vi "Handle Incoming Packets.vi"(8 "error in (no error)":errorcluster, 9 "SessionMailbox":refnum<queue>, 10 "Incoming Packet":refnum<class "ControlPacket.lvclass">, 11 "Client in":refnum<class "Client.lvclass">) -> (0 "error out":errorcluster, 1 "SessionMailbox out":refnum<queue>, 2 "Outgoing":T1, 3 "Client out":refnum<class "Client.lvclass">)   [LabVIEW 2013, in "MQTT Server.lvlib" / "Client.lvclass"]
uses:
  Client.lvclass
  Control Packets/ControlPacket/ControlPacket.lvclass
  MQTT_Base/Response -- cluster.ctl
  Client.lvclass/Client.ctl
  Control Packets/CONNACK/CONNACK.lvclass
  Control Packets/CONNACK/Connect Return Code -- enum.ctl
  MQTT_Base/MQTT_Base.lvclass
  Control Packets/PUBREC/PUBREC.lvclass
  Control Packets/ControlPacket/ControlPacket.lvclass/ControlPacket.ctl
  Control Packets/PUBLISH/PUBLISH.lvclass
  Control Packets/PUBCOMP/PUBCOMP.lvclass
  Control Packets/SUBACK/SUBACK.lvclass
  Control Packets/UNSUBACK/UNSUBACK.lvclass
  Control Packets/PINGRESP/PINGRESP.lvclass
  Control Packets/PUBREL/PUBREL.lvclass
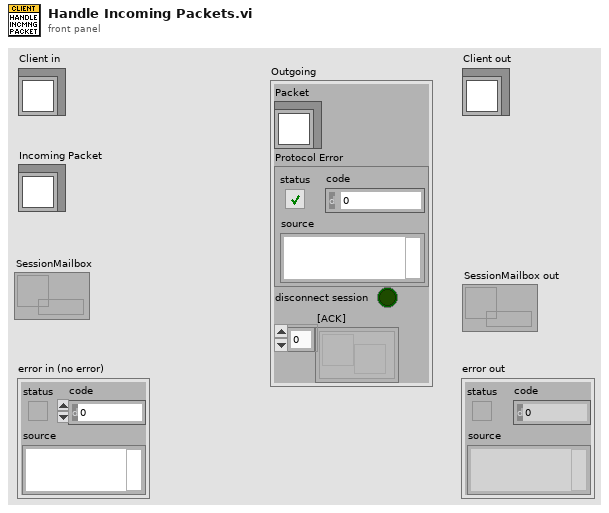
[diagram p1: front panel]
types:
  T1 = typedef "MQTT Server.lvlib/MQTT_Base.lvclass/Response -- cluster.ctl" = cluster{"Packet":refnum<class "ControlPacket.lvclass">, "Protocol Error":errorcluster, "disconnect session":bool, "[ACK]":refnum<notifier>[]}
  T2 = typedef "CONNACK.lvclass/Connect Return Code -- enum.ctl" = enum16{"Connection accepted", "Unacceptable protocol version", "Identifier Rejected", "Server Unavailable", "Bad Username or Password", "Not Authorized"}
  T3 = typedef "ControlPacket.lvclass/Control Packet Type -- enum.ctl" = enum16{"Reserved", "CONNECT", "CONNACK", "PUBLISH", "PUBACK", "PUBREC", "PUBREL", "PUBCOMP", "SUBSCRIBE", "SUBACK", "UNSUBSCRIBE", "UNSUBACK", "PINGREQ", "PINGRESP", "DISCONNECT", "Reserved(15)"}
  T4 = typedef "MQTT Server.lvlib/Client.lvclass/Public Events -- cluster.ctl" = cluster{"Connection Status":refnum<user-event>, "Connected":refnum<user-event>, "Application Message":refnum<user-event>}
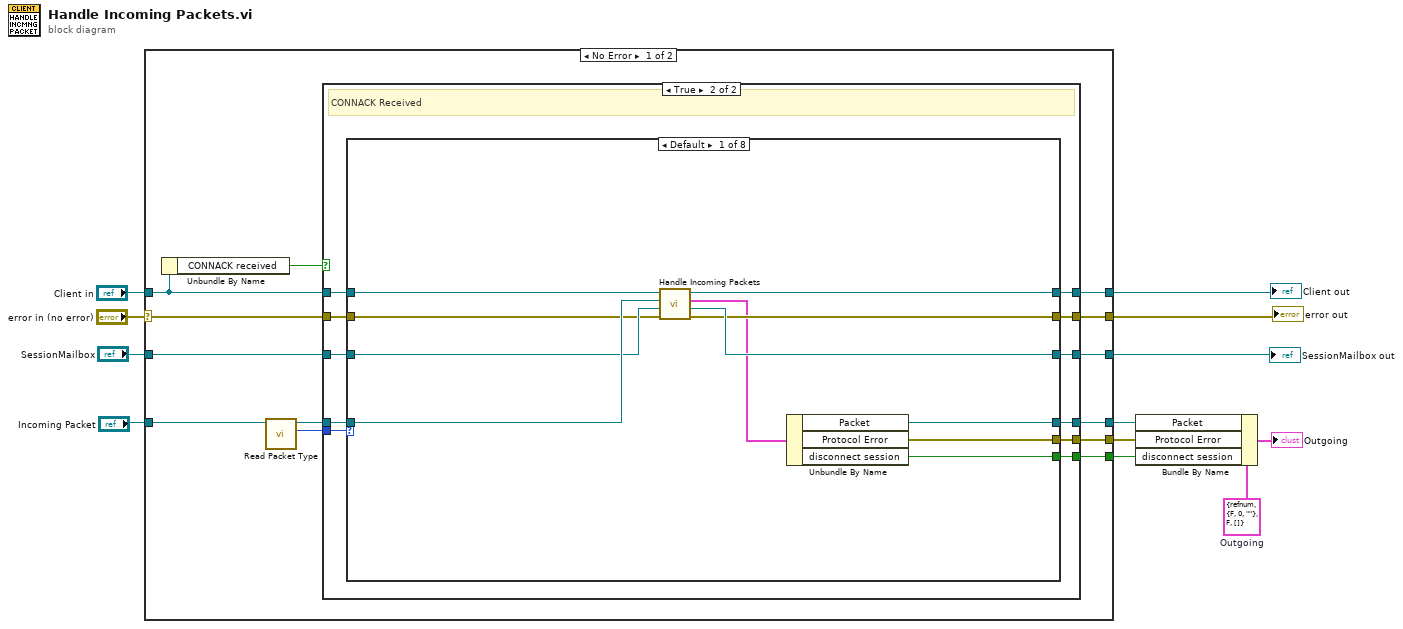
[diagram p0: block diagram]
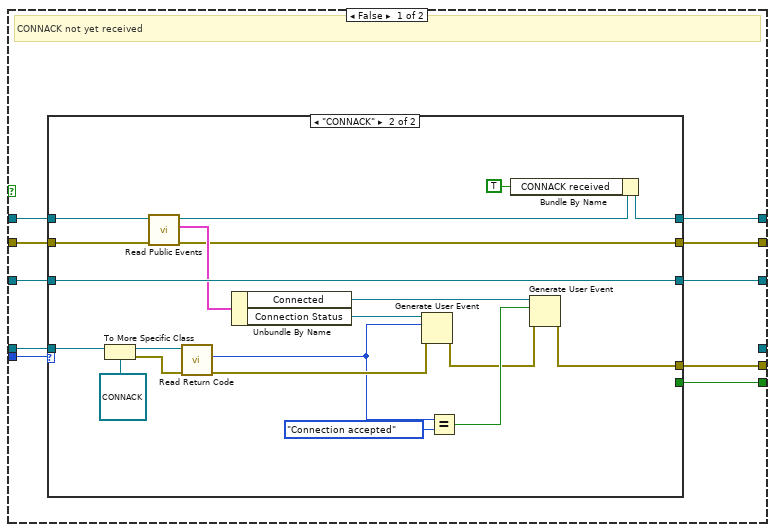
[diagram p2: hidden frame]
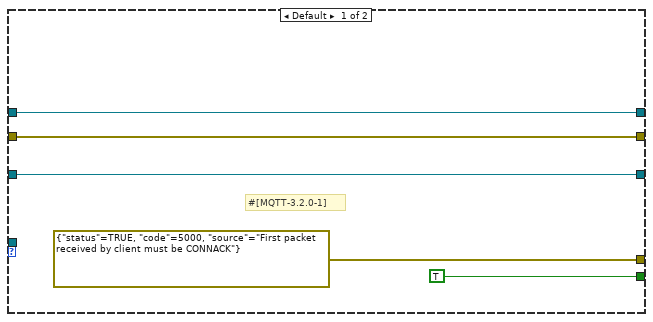
[diagram p3: hidden frame]
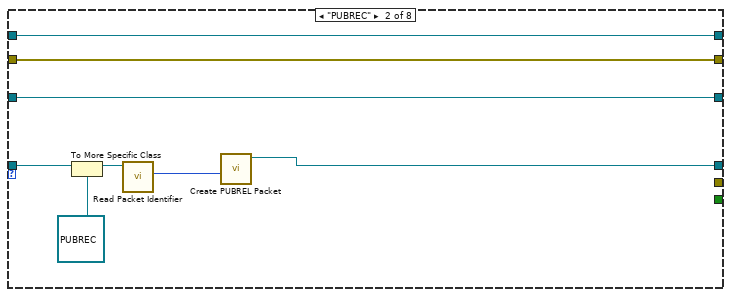
[diagram p4: hidden frame]
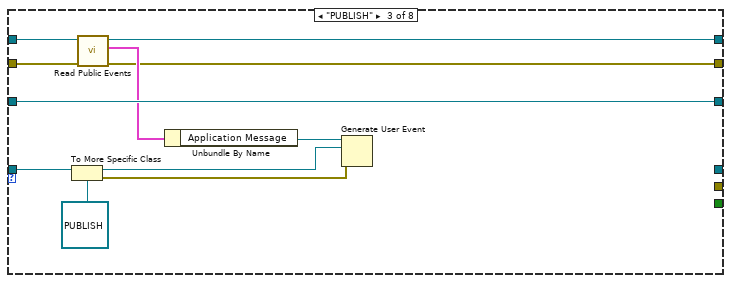
[diagram p5: hidden frame]
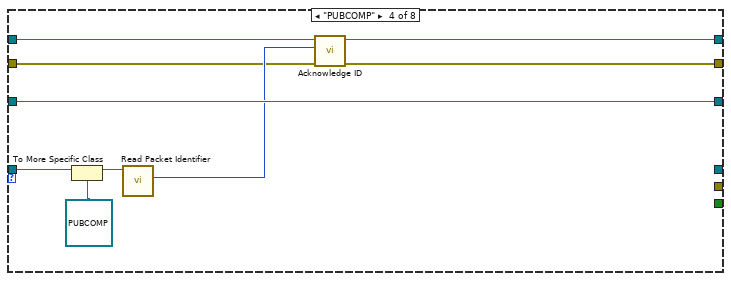
[diagram p6: hidden frame]
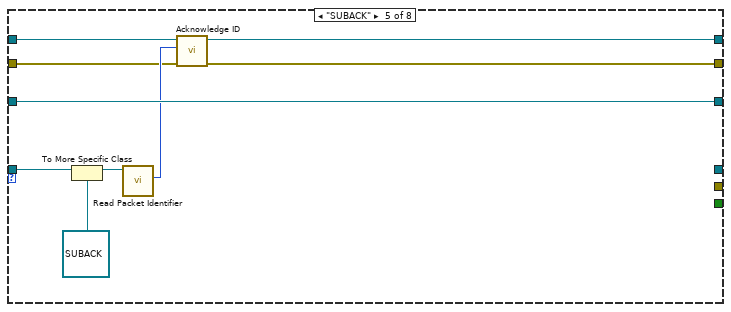
[diagram p7: hidden frame]
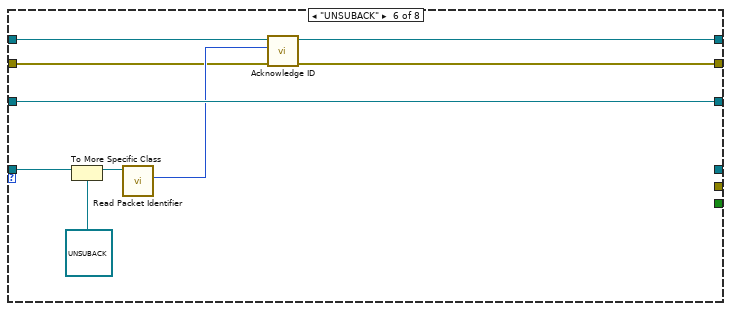
[diagram p8: hidden frame]
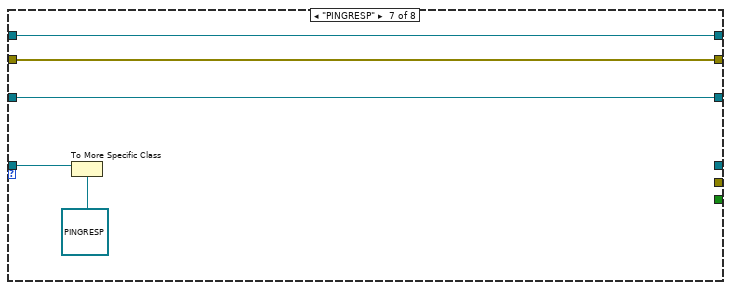
[diagram p9: hidden frame]
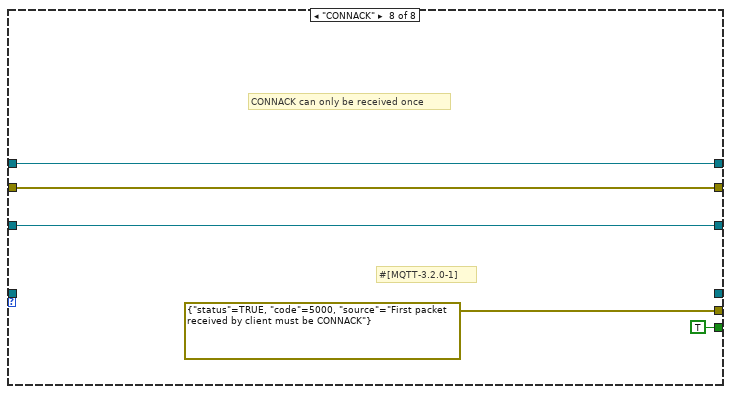
[diagram p10: hidden frame]
diagram:
  w12 = T1 {"Packet"=refnum, "Protocol Error"={"status"=FALSE, "code"=0, "source"=""}, "disconnect session"=FALSE, "[ACK]"=[]}  # Outgoing
  n1 = case shown="No Error" "error in (no error)" {
    selector: "error in (no error)" -> [w23 w141]
    tunnel: [w21 w141] -> w4
    tunnel: [w22 w140] -> w8
    tunnel: "Client in" -> [w14 w140]
    tunnel: "Incoming Packet" -> [w17 _]
    tunnel: [w20 _] -> w1
    tunnel: [w19 _] -> w10
    tunnel: "SessionMailbox" -> [w18 w139]
    tunnel: [w16 w139] -> w3
    tunnel: [w15 _] -> w11
    frame No Error {
      n2 = Unbundle By Name(w14) -> ("CONNACK received"=w13:bool)
      n3 = call "Read Packet Type.vi"("ControlPacket in"=w17) -> ("Control Packet Type"=w25:T3, "ControlPacket out"=w24:refnum<class "ControlPacket.lvclass">)  [unwired: 9 in]
      n4 = case shown="True" w13 {
        tunnel: w25 -> [w32 w71]
        tunnel: w24 -> [w35 w70]
        tunnel: w23 -> [w29 w69]
        tunnel: [w31 w68] -> w22
        tunnel: [w30 w67] -> w21
        tunnel: [_ w66] -> w20
        tunnel: [w34 w65] -> w19
        tunnel: w18 -> [w27 w64]
        tunnel: [w28 w63] -> w16
        tunnel: [w26 w62] -> w15
        tunnel: w14 -> [w33 w61]
        frame False {
          # "CONNACK not yet received"
          n5 = case shown="\"CONNACK\"" w32 {
            tunnel: w35 -> [_ w52]
            tunnel: [errorcluster {"status"=TRUE, "code"=5000, "source"="First packet received by client must be CONNACK"} ("error out 2") w51] -> w34
            tunnel: w33 -> [w40 w44]
            tunnel: [w40 w50] -> w31
            tunnel: [w39 w41] -> w30
            tunnel: w29 -> [w39 w42]
            tunnel: w27 -> [w38 w48]
            tunnel: [w38 w48] -> w28
            tunnel: [TRUE ("status") _] -> w26
            frame Default {
              # "#[MQTT-3.2.0-1]"
            }
            frame "CONNACK" {
              n6 = To More Specific Class(target class=refnum<class "CONNACK.lvclass"> refnum ("CONNACK in"), reference=w52) -> (specific class reference=w59:refnum<class "CONNACK.lvclass">, error out=w58:errorcluster)  [unwired: 1 in]
              n7 = call "Read Public Events.vi"("error in (no error)"=w42, "Client in"=w44) -> ("error out"=w41:errorcluster, "Client Public Events"=w47:T4, "Client out"=w43:refnum<class "Client.lvclass">)  [unwired: 7 in]
              n8 = call "Read Return Code.vi"("error in (no error)"=w58, "CONNACK in"=w59) -> ("error out"=w57:errorcluster, "Return Code"=w56:T2)  [unwired: 7 in, 1 out]
              n9 = Unbundle By Name(w47) -> ("Connected"=w46:refnum<user-event>, "Connection Status"=w45:refnum<user-event>)
              n10 = Generate User Event(user event=w45, event data cluster=w56, error in=w57) -> (error out=w53:errorcluster)  [unwired: 1 in, 1 out]
              n11 = Equal?(x=w56, y=Connect_Return_Code_--_enum."Connection accepted") -> (x = y?=w54:bool)
              n12 = Bundle By Name(cluster=w43, "CONNACK received"=TRUE) -> (w50:refnum<class "Client.lvclass">)
              n13 = Generate User Event(user event=w46, event data cluster=w54, error in=w53) -> (error out=w51:errorcluster)  [unwired: 1 in, 1 out]
            }
          }
        }
        frame True {
          # "CONNACK Received"
          n14 = case shown="Default" w71 {
            tunnel: w70 -> [w82 w87 w100 w109 w118 w127 w130 _]
            tunnel: w69 -> [w77 w89 w94 w103 w114 w121 w132 w138]
            tunnel: w61 -> [w79 w90 w92 w106 w112 w123 w133 w136]
            tunnel: [w78 w90 w91 w105 w111 w122 w133 w136] -> w68
            tunnel: [w76 w89 w93 w102 w113 w120 w132 w138] -> w67
            tunnel: w64 -> [w81 w88 w101 w110 w119 w128 w131 w137]
            tunnel: [w74 w83 _ _ _ _ _ _] -> w66
            tunnel: [w73 _ _ _ _ _ _ errorcluster {"status"=TRUE, "code"=5000, "source"="First packet received by client must be CONNACK"} ("error out 2")] -> w65
            tunnel: [w80 w88 w101 w110 w119 w128 w131 w137] -> w63
            tunnel: [w72 _ _ _ _ _ _ TRUE ("disconnect")] -> w62
            frame Default {
              n15 = call-parent "Handle Incoming Packets.vi"("error in (no error)"=w77, "SessionMailbox"=w81, "Incoming Packet"=w82, "MQTT_Base in"=w79) -> ("error out"=w76:errorcluster, "SessionMailbox out"=w80:refnum<queue>, "Outgoing"=w75:T1, "MQTT_Base out"=w78:refnum<class "Client.lvclass">)  [unwired: 4 in]
              n16 = Unbundle By Name(w75) -> ("Packet"=w74:refnum<class "ControlPacket.lvclass">, "Protocol Error"=w73:errorcluster, "disconnect session"=w72:bool)
            }
            frame "PUBREC" {
              n17 = To More Specific Class(target class=refnum<class "PUBREC.lvclass"> refnum ("PUBREC.lvclass"), reference=w87) -> (specific class reference=w85:refnum<class "PUBREC.lvclass">)  [unwired: 1 in, 1 out]
              n18 = call "Read Packet Identifier.vi"("ControlPacket in"=w85) -> ("Packet Identifier"=w84:u16)  [unwired: 9 in, 1 out]
              n19 = call "Create PUBREL Packet.vi"("Packet ID"=w84) -> ("PUBREL out"=w83:refnum<class "PUBREL.lvclass">)  [unwired: 9 in, 1 out]
            }
            frame "PUBLISH" {
              n20 = To More Specific Class(target class=refnum<class "PUBLISH.lvclass"> refnum ("PUBLISH.lvclass"), reference=w100) -> (specific class reference=w96:refnum<class "PUBLISH.lvclass">, error out=w95:errorcluster)  [unwired: 1 in]
              n21 = call "Read Public Events.vi"("error in (no error)"=w94, "Client in"=w92) -> ("error out"=w93:errorcluster, "Client Public Events"=w98:T4, "Client out"=w91:refnum<class "Client.lvclass">)  [unwired: 7 in]
              n22 = Unbundle By Name(w98) -> ("Application Message"=w97:refnum<user-event>)
              n23 = Generate User Event(user event=w97, event data cluster=w96, error in=w95) -> ()  [unwired: 1 in, 2 out]
            }
            frame "PUBCOMP" {
              n24 = To More Specific Class(target class=refnum<class "PUBCOMP.lvclass"> refnum ("PUBCOMP.lvclass"), reference=w109) -> (specific class reference=w108:refnum<class "PUBCOMP.lvclass">)  [unwired: 1 in, 1 out]
              n25 = call "Read Packet Identifier.vi"("ControlPacket in"=w108) -> ("Packet Identifier"=w104:u16)  [unwired: 9 in, 1 out]
              n26 = call "Acknowledge ID.vi"("error in (no error)"=w103, "Packet Identifier"=w104, "Client in"=w106) -> ("error out"=w102:errorcluster, "Client out"=w105:refnum<class "Client.lvclass">)  [unwired: 7 in]
            }
            frame "SUBACK" {
              n27 = To More Specific Class(target class=refnum<class "SUBACK.lvclass"> refnum ("SUBACK.lvclass"), reference=w118) -> (specific class reference=w117:refnum<class "SUBACK.lvclass">)  [unwired: 1 in, 1 out]
              n28 = call "Read Packet Identifier.vi"("ControlPacket in"=w117) -> ("Packet Identifier"=w115:u16)  [unwired: 9 in, 1 out]
              n29 = call "Acknowledge ID.vi"("error in (no error)"=w114, "Packet Identifier"=w115, "Client in"=w112) -> ("error out"=w113:errorcluster, "Client out"=w111:refnum<class "Client.lvclass">)  [unwired: 7 in]
            }
            frame "UNSUBACK" {
              n30 = To More Specific Class(target class=refnum<class "UNSUBACK.lvclass"> refnum ("UNSUBACK.lvclass"), reference=w127) -> (specific class reference=w126:refnum<class "UNSUBACK.lvclass">)  [unwired: 1 in, 1 out]
              n31 = call "Read Packet Identifier.vi"("ControlPacket in"=w126) -> ("Packet Identifier"=w124:u16)  [unwired: 9 in, 1 out]
              n32 = call "Acknowledge ID.vi"("error in (no error)"=w121, "Packet Identifier"=w124, "Client in"=w123) -> ("error out"=w120:errorcluster, "Client out"=w122:refnum<class "Client.lvclass">)  [unwired: 7 in]
            }
            frame "PINGRESP" {
              n33 = To More Specific Class(target class=refnum<class "PINGRESP.lvclass"> refnum ("PINGRESP.lvclass"), reference=w130) -> ()  [unwired: 1 in, 2 out]
            }
            frame "CONNACK" {
              # "#[MQTT-3.2.0-1]"
              # "CONNACK can only be received once"
            }
          }
        }
      }
    }
    frame Error {
    }
  }
  "error out" <- w4
  "Client out" <- w8
  "SessionMailbox out" <- w3
  n34 = Bundle By Name(cluster=w12, "Packet"=w1, "Protocol Error"=w10, "disconnect session"=w11) -> (→"Outgoing":T1)
